vi "Meas Asynchronous Wait.vi"(5 "Allow hard kill? (True)":bool=TRUE, 7 "Wait for exit? (False)":bool, 8 "error in":errorcluster, 9 "Force kill (False)":bool, 10 "stop button name ('btn stop')":string="btn stop", 11 "VI reference (empty)":refnum<vi>) -> (0 "error out":errorcluster, 1 "VI's error out":errorcluster, 2 "VI returned?":bool, 3 "parameter out":variant, 4 "VI exited?":bool)   [LabVIEW 2018]
doc: "This will check state of asynchronously called VI (or wait for its exit if requested). In the check only mode ('Wait for exit?' = False) it will test if the VI exited with zero timeout. If it did, it will return 'VI returned?' = True and the content of 'VI's error out' and 'parameter out' will be valid. Flag 'VI exited?' will be true whenever VI exited or VI reference is invalid.\nIn the wait mode ('Wait for exit?' = True) it will first signalize to stop by setting boolean variable named by control 'stop button name' to True (requires the SGUI library and the variable reference must be registered). Then it waits for 10s to VI exit. If it does not exit it may try to kill it (must be allowed by 'Allow hard kill?' = True). If it won't exit even after that it will return error on 'error out'. Otherwise the error out is always just a copy of input error.\nNote that this VI can return 'VI returned?' flag True only once! So when you request returned data always check the flag and if True, capture the outputs."
uses:
  varilib/varilib.lvlib
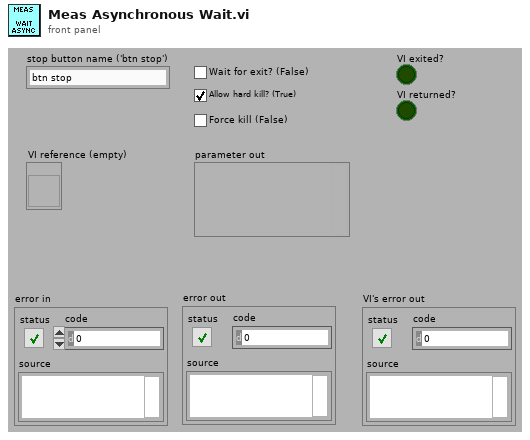
[diagram p1: front panel]
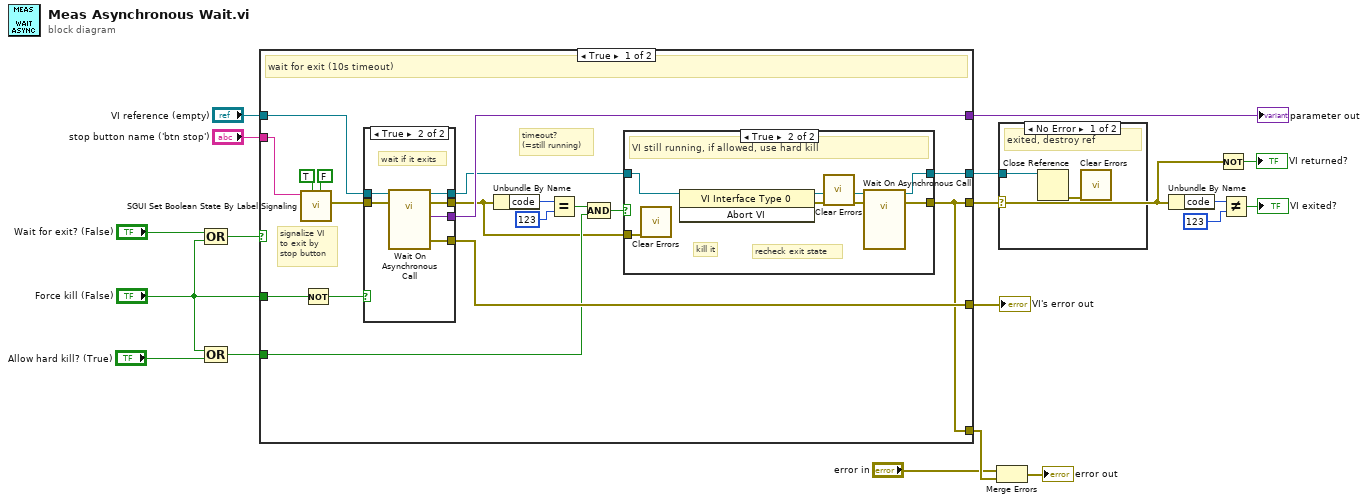
[diagram p0: block diagram]
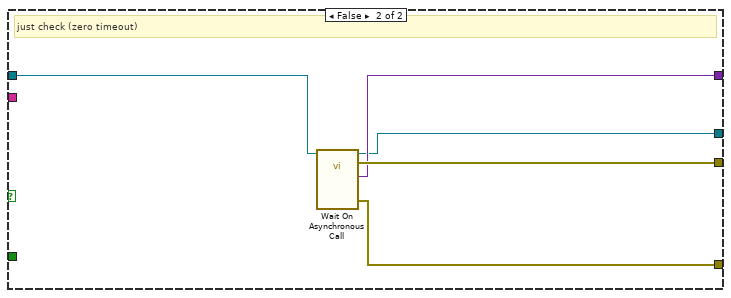
[diagram p5: hidden frame]
diagram:
  n1 = Compound Arithmetic op=OR("Wait for exit? (False)", "Force kill (False)") -> (w4:bool)
  n2 = Compound Arithmetic op=OR("Force kill (False)", "Allow hard kill? (True)") -> (w3:bool)
  n3 = case shown="True" w4 {
    tunnel: "VI reference (empty)" -> [w34 w58]
    tunnel: [w25 w57] -> w9
    tunnel: [w36 w56] -> w11
    tunnel: [w35 w55] -> w16
    tunnel: "stop button name ('btn stop')" -> [w21 _]
    tunnel: w3 -> [w28 _]
    tunnel: [w26 w54] -> w15
    tunnel: [w25 _] -> w8
    tunnel: "Force kill (False)" -> [w19 _]
    frame True {
      # "timeout?\n(=still running)"
      # "signalize VI\nto exit by\nstop button"
      # "wait for exit (10s timeout)"
      n4 = call "SGUI Set Boolean State By Label Signaling.vi"("generate error if not found? (True)"=FALSE, "binary state in (False)"=TRUE, "control label(s) ('btn stop')"=w21) -> ("error out"=w24:errorcluster)  [unwired: 7 in, 1 out]
      n5 = Not(x=w19) -> (.not. x?=w20:bool)
      n6 = case shown="True" w20 {
        tunnel: [_ w44] -> w36
        tunnel: [_ w43] -> w35
        tunnel: w34 -> [w37 w42]
        tunnel: [w37 w41] -> w33
        tunnel: [w38 w40] -> w27
        tunnel: w24 -> [w38 w39]
        frame False {
        }
        frame True {
          # "wait if it exits"
          n7 = call-by-ref "Wait On Asynchronous Call"(reference=w42, error in=w39) -> (reference out=w41:refnum<vi>, error out=w40:errorcluster, 0:"error out"=w44:errorcluster, "aux data out"=w43:variant)  [unwired: 10 in]
        }
      }
      n8 = Unbundle By Name(w27) -> ("code"=w32:i32)
      n9 = Equal?(x=w32, y=123) -> (x = y?=w30:bool)
      n10 = Compound Arithmetic op=AND(w30, w28) -> (w29:bool)
      n11 = case shown="True" w29 {
        tunnel: [w46 w51] -> w25
        tunnel: w33 -> [w45 w53]
        tunnel: w27 -> [w46 w47]
        tunnel: [w45 w48] -> w26
        frame False {
        }
        frame True {
          # "recheck exit state"
          # "kill it"
          # "VI still running, if allowed, use hard kill"
          n12 = call <vilib>:"Clear Errors.vi"("error in (no error)"=w47) -> ()  [unwired: 5 in, 2 out]
          n13 = invoke class="VI Interface Type 0" method="Abort VI"(reference=w53) -> (reference out=w52:refnum<vi>, error out=w50:errorcluster)  [unwired: 2 in, 1 out]
          n14 = call <vilib>:"Clear Errors.vi"("error in (no error)"=w50) -> ("error out"=w49:errorcluster)  [unwired: 5 in, 1 out]
          n15 = call-by-ref "Wait On Asynchronous Call"(reference=w52, error in=w49) -> (reference out=w48:refnum<vi>, error out=w51:errorcluster)  [unwired: 10 in, 2 out]
        }
      }
    }
    frame False {
      # "just check (zero timeout)"
      n16 = call-by-ref "Wait On Asynchronous Call"(reference=w58) -> (reference out=w54:refnum<vi>, error out=w57:errorcluster, 0:"error out"=w56:errorcluster, "aux data out"=w55:variant)  [unwired: 11 in]
    }
  }
  "parameter out" <- w16
  "VI's error out" <- w11
  n17 = Merge Errors("error in", w8) -> (→"error out":errorcluster)
  n18 = case shown="No Error" w9 {
    tunnel: w15 -> [w60 _]
    frame No Error {
      # "exited, destroy ref"
      n19 = Close Reference(reference=w60) -> (error out=w59:errorcluster)  [unwired: 1 in]
      n20 = call <vilib>:"Clear Errors.vi"("error in (no error)"=w59) -> ()  [unwired: 5 in, 2 out]
    }
    frame Error {
      # "still running?\ndo nothing"
    }
  }
  n21 = Unbundle By Name(w9) -> ("code"=w14:i32)
  n22 = Not(x=w9) -> (.not. x?=→"VI returned?":bool)
  n23 = Not Equal?(x=w14, y=123) -> (x != y?=→"VI exited?":bool)
